vi "Log CodeGen Run.vi"(8 "error In":errorcluster, 11 "To Generate":enum16{"gRPC Server", "gRPC Client", "Both"}(ring)) -> (0 "error out":errorcluster)   [LabVIEW 2019, in "gRPC Template Creation Utility.lvlib"]
uses:
  gRPC Template Creation Utility.lvlib
  <vilib>/UDC/Controls/LogMessageFrequency.ctl
  <vilib>/UDC/niceiplib.lvlib
  <vilib>/UDC/Controls/LogMessageSize.ctl
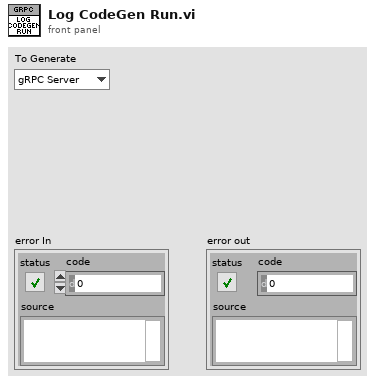
[diagram p1: front panel]
types:
  T1 = typedef "niceiplib.lvlib/LogMessageSize.ctl" = enum32{"SmallMessage", "MediumMessage", "LargeMessage"}
  T2 = typedef "niceiplib.lvlib/LogMessageFrequency.ctl" = enum32{"OncePerSession", "LowFrequency", "MediumFrequency", "HighFrequency", "KBMouseEvents"}
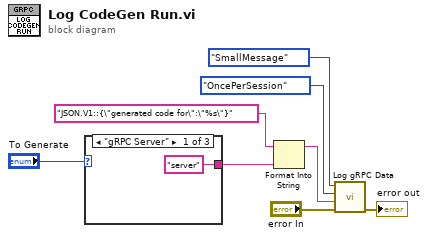
[diagram p0: block diagram]
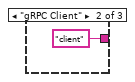
[diagram p2: hidden frame]
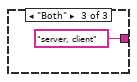
[diagram p3: hidden frame]
diagram:
  n1 = case shown="\"gRPC Server\"" "To Generate" {
    tunnel: ["server" "client" "server, client"] -> w2
    frame "gRPC Server" {
    }
    frame "gRPC Client" {
    }
    frame "Both" {
    }
  }
  n2 = Format Into String(initial string="JSON.V1::{\"generated code for\":\"%s\"}", w2) -> (resulting string=w1:string)  [unwired: 2 in, 1 out]
  n3 = call "Log gRPC Data.vi"("error in (no error)"="error In", "Value"=w1, "LogMessageFrequency"=LogMessageFrequency."OncePerSession", "LogMessageSize"=LogMessageSize."SmallMessage") -> ("error out"=→"error out":errorcluster)  [unwired: 7 in]
